vi "SSC DAQmx Calculate Per-Instrument to Per-Site Per-Pin LUT.vi"(0 "DAQmx SSC in":T1[](array[typedef]), 7 "Sites":i32[](array[numeric]), 9 "Pins":string[](array[string])) -> (4 "Per-Task to Per-Site Per-Pin LUT":T2[](array[typedef]))   [LabVIEW 2020]
uses:
  Digital/SubVIs/Digital 2D Location Array in a Cluster.ctl
  Digital/SubVIs/Digital 2D Location.ctl
  Pin Map/SSC DAQmx.ctl
  Shared SubVIs/Trim Whitespace [Inlined].vi
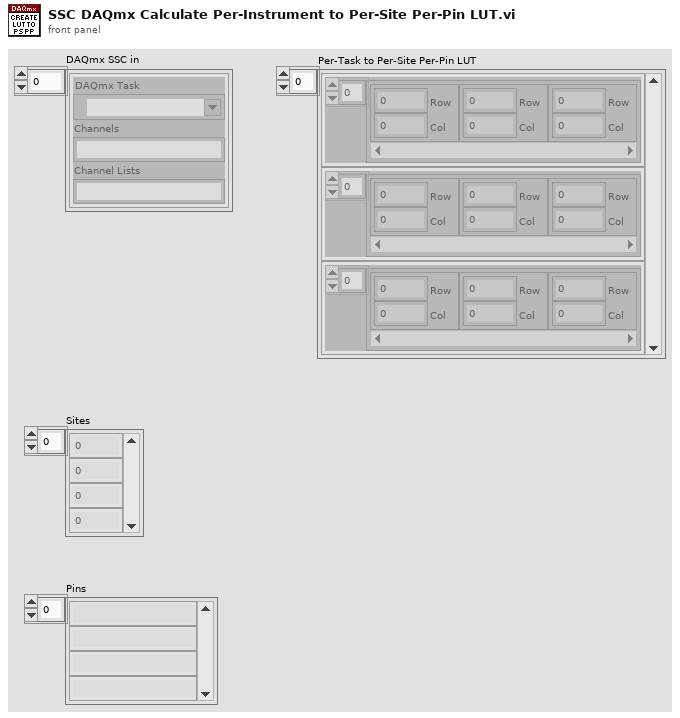
[diagram p1: front panel]
types:
  T1 = typedef "SSC DAQmx.ctl" = cluster{"DAQmx Task ":refnum<k21>, "Channels":string, "Channel Lists":string}
  T2 = typedef "Digital 2D Location Array in a Cluster.ctl" = cluster{"Digital 2D Location Array":T3[]}
  T3 = typedef "Digital 2D Location.ctl" = cluster{"Row":i32, "Col":i32}
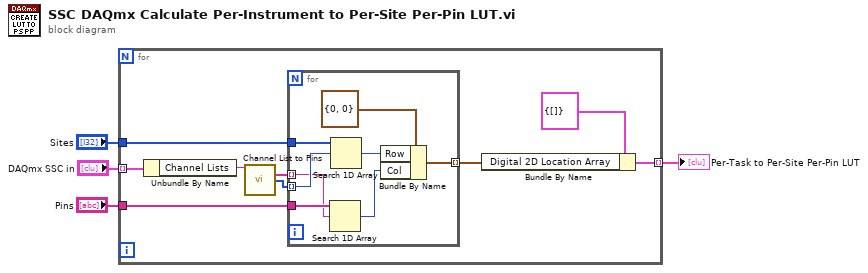
[diagram p0: block diagram]
diagram:
  n1 = for {
    tunnel: "DAQmx SSC in" -> [w13] mode=indexing
    tunnel: "Sites" -> [w8]
    tunnel: "Pins" -> [w9]
    tunnel: [w6] -> w2 mode=indexing
    n2 = Unbundle By Name(w13) -> ("Channel Lists"=w12:string)
    n3 = call "Channel List to Pins.vi"("Channel List"=w12) -> ("Pins"=w11:tag[], "Sites"=w10:i32[])  [unwired: 12 in, 1 out]
    n4 = for {
      tunnel: w11 -> [w18] mode=indexing
      tunnel: w10 -> [w20] mode=indexing
      tunnel: w9 -> [w19]
      tunnel: w8 -> [w21]
      tunnel: [w17] -> w7 mode=indexing
      n5 = Search 1D Array(1D array=w19, element=w18) -> (index of element=w15:i32)  [unwired: 1 in]
      n6 = Search 1D Array(1D array=w21, element=w20) -> (index of element=w16:i32)  [unwired: 1 in]
      n7 = Bundle By Name(cluster=T3 {"Row"=0, "Col"=0}, "Row"=w16, "Col"=w15) -> (w17:T3)
    }
    n8 = Bundle By Name(cluster=T2 {"Digital 2D Location Array"=[]} ("Digital 2D Location Array in a Cluster"), "Digital 2D Location Array"=w7) -> (w6:T2)
  }
  "Per-Task to Per-Site Per-Pin LUT" <- w2
